vi "Measurement.PhotocurrentMapping.GetStaticDependencies.vi"(8 "error in (no error)":errorcluster, 11 "Measurement.PhotocurrentMapping in":refnum<class "Measurement.PhotocurrentMapping.lvclass">) -> (0 "error out":errorcluster, 2 "Dependencies":T1, 3 "Measurement.PhotocurrentMapping out":refnum<class "Measurement.PhotocurrentMapping.lvclass">)   [LabVIEW 2017, in "Measurement.PhotocurrentMapping.lvclass"]
uses:
  Measurement.PhotocurrentMapping.lvclass
  D:/Program Files (x86)/National Instruments/LabVIEW 2017/vi.lib/JKI/JKI SMO/SMO/SMO.lvclass
  Typedefs/Dependencies--Cluster.ctl
  SMU/SMU.lvclass
  LIA/LIA.lvclass
  XYStage/XYStage.lvclass
  <vilib>/JKI/JKI SMO/SMO/SMO.lvclass
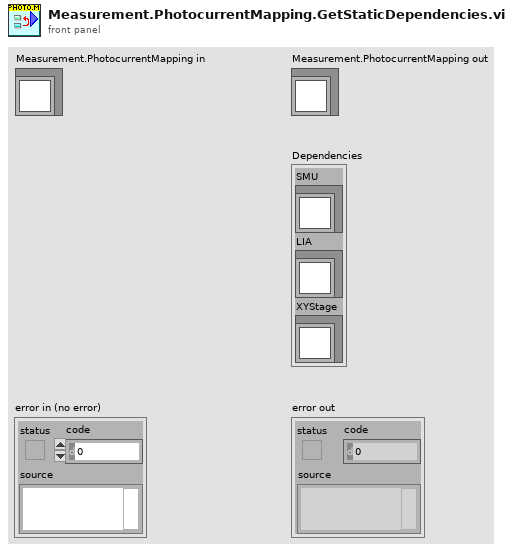
[diagram p1: front panel]
types:
  T1 = typedef "Measurement.PhotocurrentMapping.lvclass/Dependencies--Cluster.ctl" = cluster{"SMU":refnum<class "SMU.lvclass">, "LIA":refnum<class "LIA.lvclass">, "XYStage":refnum<class "XYStage.lvclass">}
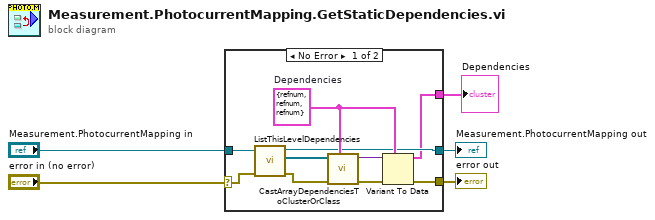
[diagram p0: block diagram]
diagram:
  n1 = case shown="No Error" "error in (no error)" {
    selector: "error in (no error)" -> [w14 w17]
    tunnel: [w8 w17] -> w4
    tunnel: [w7 w16] -> w2
    tunnel: "Measurement.PhotocurrentMapping in" -> [w15 w16]
    tunnel: [w6 _] -> w1
    frame No Error {
      w9 = T1 {"SMU"=refnum, "LIA"=refnum, "XYStage"=refnum}  # Dependencies
      n2 = call <vilib>:"ListThisLevelDependencies.vi"("error in (no error)"=w14, "SMO in"=w15) -> ("error out"=w12:errorcluster, "[My Dependencies]"=w13:refnum<class "SMO.lvclass">[], "SMO out"=w7:refnum<class "Measurement.PhotocurrentMapping.lvclass">)  [unwired: 7 in]
      n3 = call <vilib>:"CastArrayDependenciesToClusterOrClass.vi"("Dependency Type (Class|Cluster)"=w9, "error in (no error)"=w12, "[Dependencies]"=w13) -> ("error out"=w11:errorcluster, "Dependencies output"=w10:variant)  [unwired: 7 in]
      n4 = Variant To Data(error in=w11, type=w9, Variant=w10) -> (data=w6:T1, error out=w8:errorcluster)
    }
    frame Error {
    }
  }
  "error out" <- w4
  "Measurement.PhotocurrentMapping out" <- w2
  "Dependencies" <- w1
